vi "Configure Recording.vi"(8 "error in (no error)":errorcluster, 9 "Max number of frames":dbl=10000.0 format="%#_13g", 10 "Rigid Body":T1, 11 "Frame Grabber Data In":T4={"Camera Session"="", "Frame"=refnum, "AVI Refnum"=refnum, "Codecs"=[], "Frame number"=0, "Tracking File Refnum"=refnum, "Tick Count"=0, "Probe Object"=refnum, "Playback Probe Data"=[], "Rigid Body"={"Position"={"x (mm)"=0.0, "y (mm)"=0.0, "z (mm)"=0.0}, "Orientation"={"Pitch (rad)"=0.0, "Yaw (rad)"=0.0, "Roll (rad)"=0.0}, "Quaternion"={"qx"=0.0, "qy"=0.0, "qz"=0.0, "qw"=0.0}, "Tracked?"=FALSE}, "Total no frames playback"=0, "Video FPS"=0.0, "Camera connected?"=FALSE, "Scene"=refnum, "Cropped Frame"=refnum, "Tracker FPS"=0.0, "Crop ROI"=[], "Presentation Values"=[], "Elapsed time (ms)"=0, "Camera frames playback"=0, "Refnums"={"Live Refnum"=refnum, "Record Refnum"=refnum, "Recording Settings Refnum"=refnum, "Playback Refnum"=refnum, "Frame Slider Refnum"=refnum, "Pause Refnum"=refnum, "Home Refnum"=refnum, "Crop Refnum"=refnum, "Clear Crop Refnum"=refnum, "stop refnum"=refnum, "Playback Rate Refnum"=refnum, "Operator Settings Refnums"=refnum, "Presentation Refnum"=refnum, "Gestation Refnum"=refnum, "Connection Settings Refnum"=refnum, "Crop Time Frame Slider Refnum"=refnum}, "Dimensions"={"Probe Dimensions"={"Probe Width"=0.0, "Probe Depth"=1.0, "Probe Height"=0.0}, "Room Dimensions"={"Room Width"=0.0, "Room Depth"=0.0, "Room Height"=0.0}}, "Playback Data As Strings"=[], "Cropped Tracking File Refnum"=refnum, "Cropped AVI Refnum"=refnum, "Header"=[]}) -> (0 "error out":errorcluster, 3 "Frame Grabber Data Out":T4={"Camera Session"="", "Frame"=refnum, "AVI Refnum"=refnum, "Codecs"=[], "Frame number"=0, "Tracking File Refnum"=refnum, "Tick Count"=0, "Probe Object"=refnum, "Playback Probe Data"=[], "Rigid Body"={"Position"={"x (mm)"=0.0, "y (mm)"=0.0, "z (mm)"=0.0}, "Orientation"={"Pitch (rad)"=0.0, "Yaw (rad)"=0.0, "Roll (rad)"=0.0}, "Quaternion"={"qx"=0.0, "qy"=0.0, "qz"=0.0, "qw"=0.0}, "Tracked?"=FALSE}, "Total no frames playback"=0, "Video FPS"=0.0, "Camera connected?"=FALSE, "Scene"=refnum, "Cropped Frame"=refnum, "Tracker FPS"=0.0, "Crop ROI"=[], "Presentation Values"=[], "Elapsed time (ms)"=0, "Camera frames playback"=0, "Refnums"={"Live Refnum"=refnum, "Record Refnum"=refnum, "Recording Settings Refnum"=refnum, "Playback Refnum"=refnum, "Frame Slider Refnum"=refnum, "Pause Refnum"=refnum, "Home Refnum"=refnum, "Crop Refnum"=refnum, "Clear Crop Refnum"=refnum, "stop refnum"=refnum, "Playback Rate Refnum"=refnum, "Operator Settings Refnums"=refnum, "Presentation Refnum"=refnum, "Gestation Refnum"=refnum, "Connection Settings Refnum"=refnum, "Crop Time Frame Slider Refnum"=refnum}, "Dimensions"={"Probe Dimensions"={"Probe Width"=0.0, "Probe Depth"=1.0, "Probe Height"=0.0}, "Room Dimensions"={"Room Width"=0.0, "Room Depth"=0.0, "Room Height"=0.0}}, "Playback Data As Strings"=[], "Cropped Tracking File Refnum"=refnum, "Cropped AVI Refnum"=refnum, "Header"=[]})   [LabVIEW 2017]
uses:
  Controls/Frame Grabber Data.ctl
  <vilib>/userdefined/High Color/IMAQdx.ctl
  <vilib>/vision/Image Controls.llb/IMAQ Image.ctl
  <vilib>/vision/Avi.llb/IMAQ AVI2 Refnum.ctl
  Controls/Rigid Body Info.ctl
  Controls/Position.ctl
  Controls/Orientation.ctl
  Controls/Refnums.ctl
  Controls/Recording Settings.ctl
  Controls/Operator Settings.ctl
  Controls/Operator.ctl
  Controls/Dimensions.ctl
  Controls/Room Dimensions.ctl
  <vilib>/vision/driver/NI_Vision_Acquisition_Software.lvlib
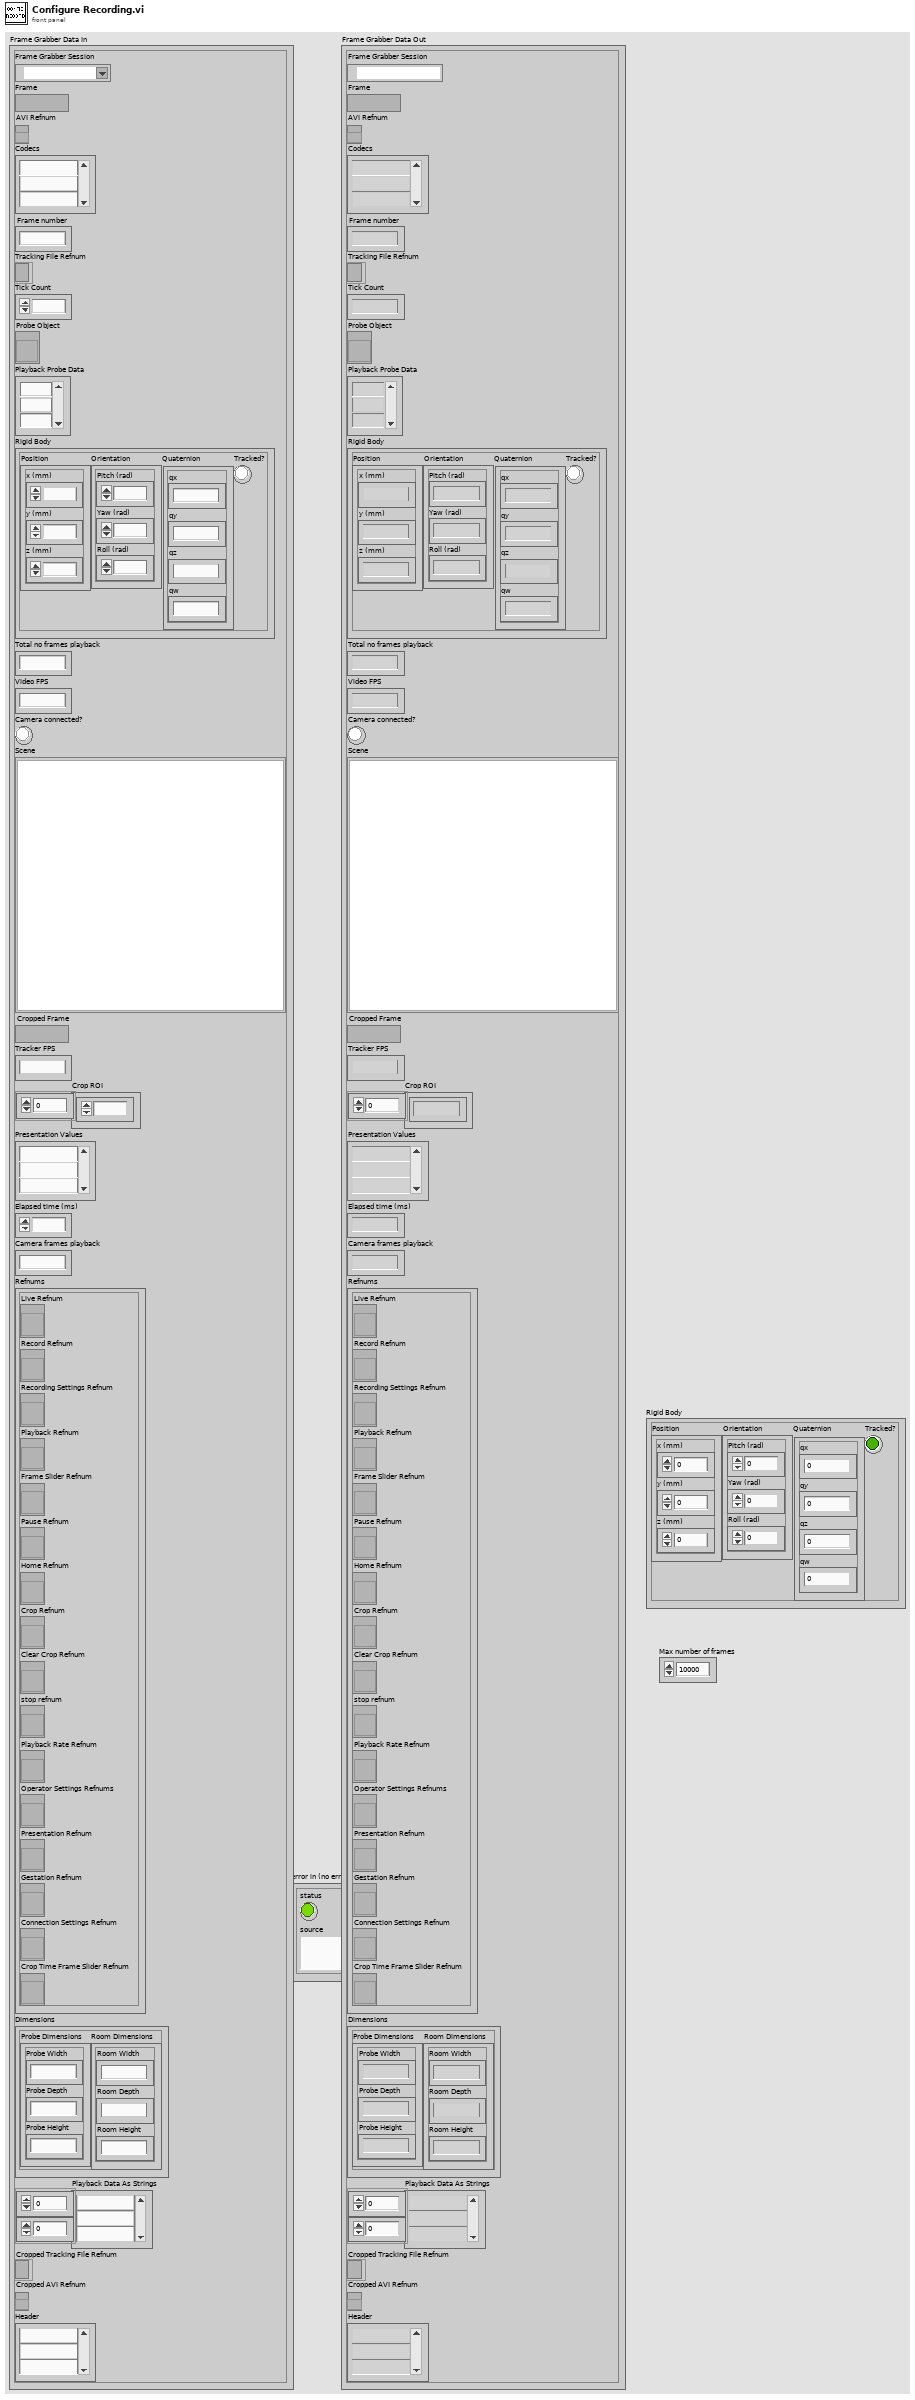
[diagram p1: front panel]
types:
  T1 = typedef "Rigid Body Info.ctl" = cluster{"Position":T2, "Orientation":T3, "Quaternion":cluster{"qx":sgl, "qy":sgl, "qz":sgl, "qw":sgl}, "Tracked?":bool}
  T2 = typedef "Position.ctl" = cluster{"x (mm)":sgl, "y (mm)":sgl, "z (mm)":sgl}
  T3 = typedef "Orientation.ctl" = cluster{"Pitch (rad)":sgl, "Yaw (rad)":sgl, "Roll (rad)":sgl}
  T4 = typedef "Frame Grabber Data.ctl" = cluster{"Camera Session":T5, "Frame":T6, "AVI Refnum":T7, "Codecs":string[], "Frame number":u32, "Tracking File Refnum":refnum<file>, "Tick Count":u32, "Probe Object":refnum<vi>, "Playback Probe Data":dbl[][], "Rigid Body":T1, "Total no frames playback":i32, "Video FPS":dbl, "Camera connected?":bool, "Scene":refnum<vi>, "Cropped Frame":T6, "Tracker FPS":dbl, "Crop ROI":i32[], "Presentation Values":string[], "Elapsed time (ms)":u32, "Camera frames playback":u32, "Refnums":T8, "Dimensions":T9, "Playback Data As Strings":string[][], "Cropped Tracking File Refnum":refnum<file>, "Cropped AVI Refnum":T7, "Header":string[]}
  T5 = typedef "IMAQdx.ctl" = refnum<k21>
  T6 = typedef "IMAQ Image.ctl" = refnum<image>
  T7 = typedef "IMAQ AVI2 Refnum.ctl" = refnum<k20>
  T8 = typedef "Refnums.ctl" = cluster{"Live Refnum":refnum<vi>, "Record Refnum":refnum<vi>, "Recording Settings Refnum":refnum<vi>, "Playback Refnum":refnum<vi>, "Frame Slider Refnum":refnum<vi>, "Pause Refnum":refnum<vi>, "Home Refnum":refnum<vi>, "Crop Refnum":refnum<vi>, "Clear Crop Refnum":refnum<vi>, "stop refnum":refnum<vi>, "Playback Rate Refnum":refnum<vi>, "Operator Settings Refnums":refnum<vi>, "Presentation Refnum":refnum<vi>, "Gestation Refnum":refnum<vi>, "Connection Settings Refnum":refnum<vi>, "Crop Time Frame Slider Refnum":refnum<vi>}
  T9 = typedef "Dimensions.ctl" = cluster{"Probe Dimensions":cluster{"Probe Width":sgl, "Probe Depth":sgl, "Probe Height":sgl}, "Room Dimensions":T10}
  T10 = typedef "Room Dimensions.ctl" = cluster{"Room Width":dbl, "Room Depth":dbl, "Room Height":dbl}
  T11 = enum16{"open", "replace", "create", "open or create", "replace or create", "replace or create with confirmation"}
  T12 = typedef "Operator Settings.ctl" = cluster{"Operator ID":string, "Expertise":T13}
  T13 = typedef "Operator.ctl" = u16
  T14 = typedef "Recording Settings.ctl" = cluster{"Folder to Save Recording":path, "Recording Name":string, "Video FPS":dbl, "Codec":u16, "Tracker FPS":dbl}
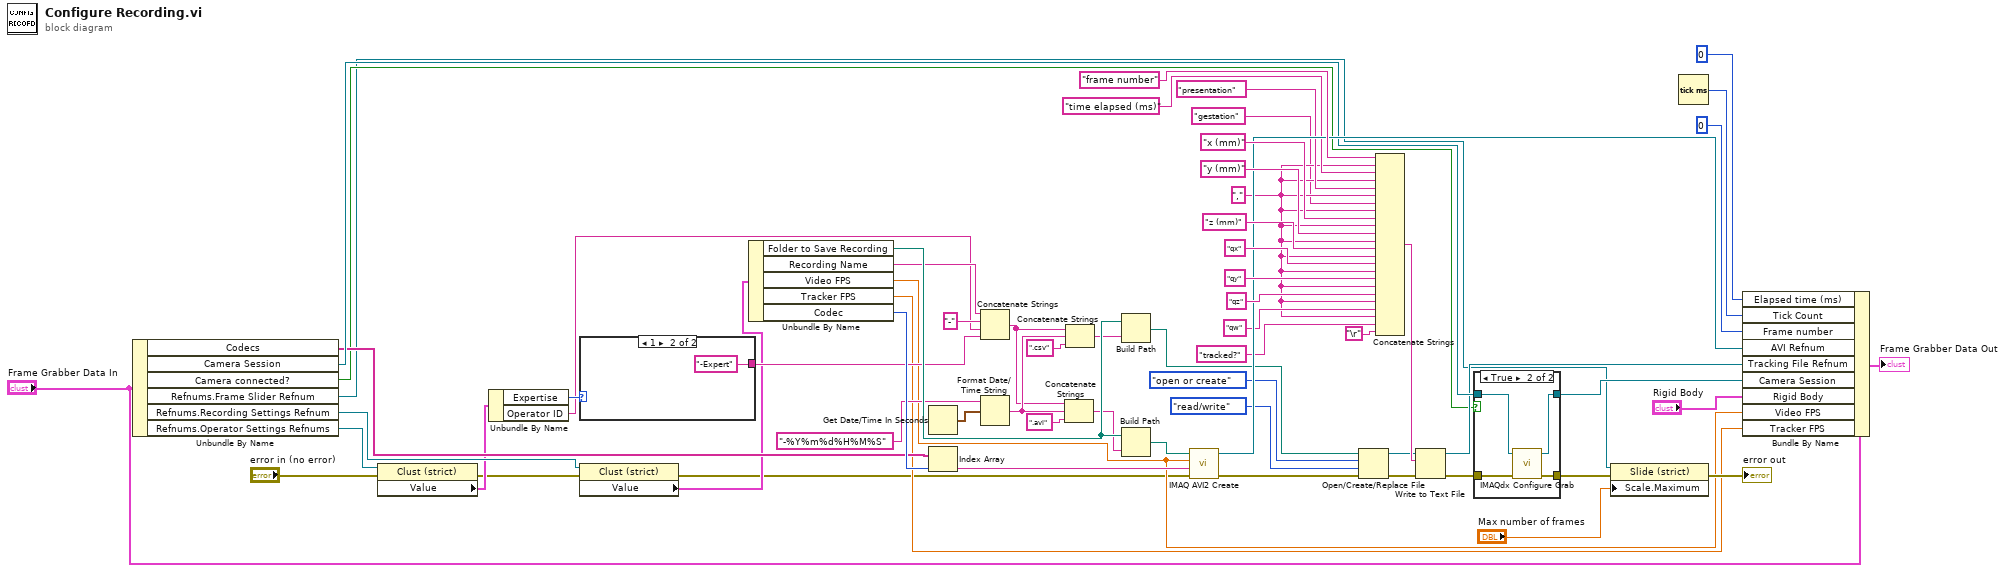
[diagram p0: block diagram]
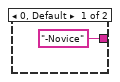
[diagram p2: hidden frame]
diagram:
  w15 = ","
  n1 = Unbundle By Name("Frame Grabber Data In") -> ("Codecs"=w40:string[], "Camera Session"=w44:T5, "Camera connected?"=w23:bool, "Refnums.Frame Slider Refnum"=w12:refnum<vi>, "Refnums.Recording Settings Refnum"=w7:refnum<vi>, "Refnums.Operator Settings Refnums"=w5:refnum<vi>)
  n2 = property class="Clust (strict)"(reference=w5, error in="error in (no error)") -> (error out=w2:errorcluster, "Value"=w4:T12)  [unwired: 1 out]
  n3 = Unbundle By Name(w4) -> ("Expertise"=w13:T13, "Operator ID"=w8:string)
  n4 = case shown="1" w13 {
    tunnel: ["-Novice" "-Expert"] -> w21
    frame 0, Default {
    }
    frame 1 {
    }
  }
  n5 = property class="Clust (strict)"(reference=w7, error in=w2) -> (error out=w1:errorcluster, "Value"=w6:T14)  [unwired: 1 out]
  n6 = Unbundle By Name(w6) -> ("Folder to Save Recording"=w52:path, "Recording Name"=w38:string, "Video FPS"=w10:dbl, "Tracker FPS"=w11:dbl, "Codec"=w53:u16)
  n7 = Get Date/Time In Seconds() -> (seconds since 1Jan1904=w42:timestamp)
  n8 = Index Array(array=w40, index=w53) -> (element=w54:string)
  n9 = Concatenate Strings(w38, "-" ("string"), w8, w21) -> (w20:string)
  n10 = Format Date/Time String(time format string (%c)="-%Y%m%d%H%M%S", seconds (now)=w42) -> (date/time string=w41:string)  [unwired: 1 in]
  n11 = Concatenate Strings(w20, w41, ".avi" ("string")) -> (w49:string)
  n12 = Concatenate Strings(w20, w41, ".csv" ("string")) -> (w50:string)
  n13 = Build Path(base path=w52, name or relative path=w50) -> (appended path=w37:path)
  n14 = Build Path(base path=w52, name or relative path=w49) -> (appended path=w39:path)
  n15 = call "IMAQ AVI2 Create"("error in (no error)"=w1, "Codec"=w54, "Frames Per Second"=w10, "AVI Path"=w39) -> ("error out"=w36:errorcluster, "AVI Refnum"=w47:T7)  [unwired: 6 in]
  n16 = Open/Create/Replace File(file path (use dialog)=w37, error in=w36, operation (0:open)=T11."open or create", access (0:read/write)=enum16{"read/write", "read-only", "write-only"}."read/write") -> (refnum out=w34:refnum<file>, error out=w35:errorcluster)  [unwired: 2 in, 1 out]
  n17 = Concatenate Strings("frame number" ("string"), w15, "time elapsed (ms)" ("string"), w15, "presentation" ("string"), w15, "gestation" ("string"), w15, "x (mm)" ("string"), w15, "y (mm)" ("string"), w15, "z (mm)" ("string"), w15, "qx" ("string"), w15, "qy" ("string"), w15, "qz" ("string"), w15, "qw" ("string"), w15, "tracked?" ("string"), "\r") -> (w64:string)
  n18 = Write to Text File(file (use dialog)=w34, text=w64, error in=w35) -> (refnum out=w33:refnum<file>, error out=w45:errorcluster)  [unwired: 1 in, 1 out]
  n19 = case shown="True" w23 {
    tunnel: w45 -> [w67 w72]
    tunnel: w44 -> [w68 w71]
    tunnel: [w68 w70] -> w27
    tunnel: [w67 w69] -> w26
    frame False {
    }
    frame True {
      n20 = call <vilib>:"IMAQdx Configure Grab.vi"("error in"=w72, "Session In"=w71) -> ("error out"=w69:errorcluster, "Session Out"=w70:T5)  [unwired: 8 in]
    }
  }
  n21 = property class="Slide (strict)"(reference=w12, error in=w26, "Scale.Maximum"="Max number of frames") -> (error out=→"error out":errorcluster)  [unwired: 1 out]
  n22 = Tick Count (ms)() -> (millisecond timer value=w30:u32)
  n23 = Bundle By Name(cluster="Frame Grabber Data In", "Elapsed time (ms)"=u32 0, "Tick Count"=w30, "Frame number"=u32 0, "AVI Refnum"=w47, "Tracking File Refnum"=w33, "Camera Session"=w27, "Rigid Body"="Rigid Body", "Video FPS"=w10, "Tracker FPS"=w11) -> (→"Frame Grabber Data Out":T4)
